vi "VMS_6_Responder.vi"() -> ()   [LabVIEW 2023]
uses:
  <vilib>/rvi/Emulation/niFpgaGetClockAttributes.vi
  <vilib>/rvi/Emulation/niFpgaSctlEmulationGetInTimedLoop.vi
  <vilib>/rvi/Emulation/niFpgaEmulationReportErrorSimple.vi
  <vilib>/rvi/eio/common/nirviEmuTemplateMethod_errors.vi
  <vilib>/eio/utilities/niEioResolveVilibRelativePath.vi
  <vilib>/rvi/interface/RandomDataEmulation/niFpgaRandomDataHandleErrors.vi
  <vilib>/rvi/Emulation/niFpgaProcessEmulError.vi
  <vilib>/rvi/Emulation/niFpgaCriticalErrorInLSC.vi
  <vilib>/rvi/occurrence/nirviWaitOnOccurrenceBase.vi
  <vilib>/eio/EIOMethodNode/EIOMethodNode.xnode
  <vilib>/rvi/DataTransferAndStorage/Container/XNode/niFpgaContainer.xnode
  <vilib>/rvi/interface/RandomDataEmulation/nirviRandomDataFpgaReadWriteTemplate.vi
  <vilib>/eio/EIONode/EIONode.xnode
panel:
  out "Ready":bool
  out "Timeouted":bool
  in  "Period (ms)":u32=5
  out "FIFO full":bool
  out "Stopped":bool
  out "Chassis Temperature":fxp<+/-,32,16>
  out "Ticks":u64
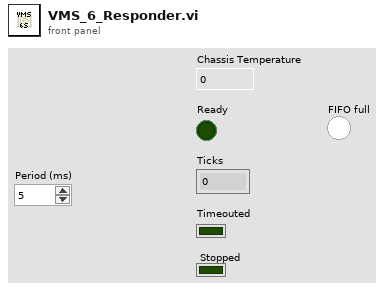
[diagram p1: front panel]
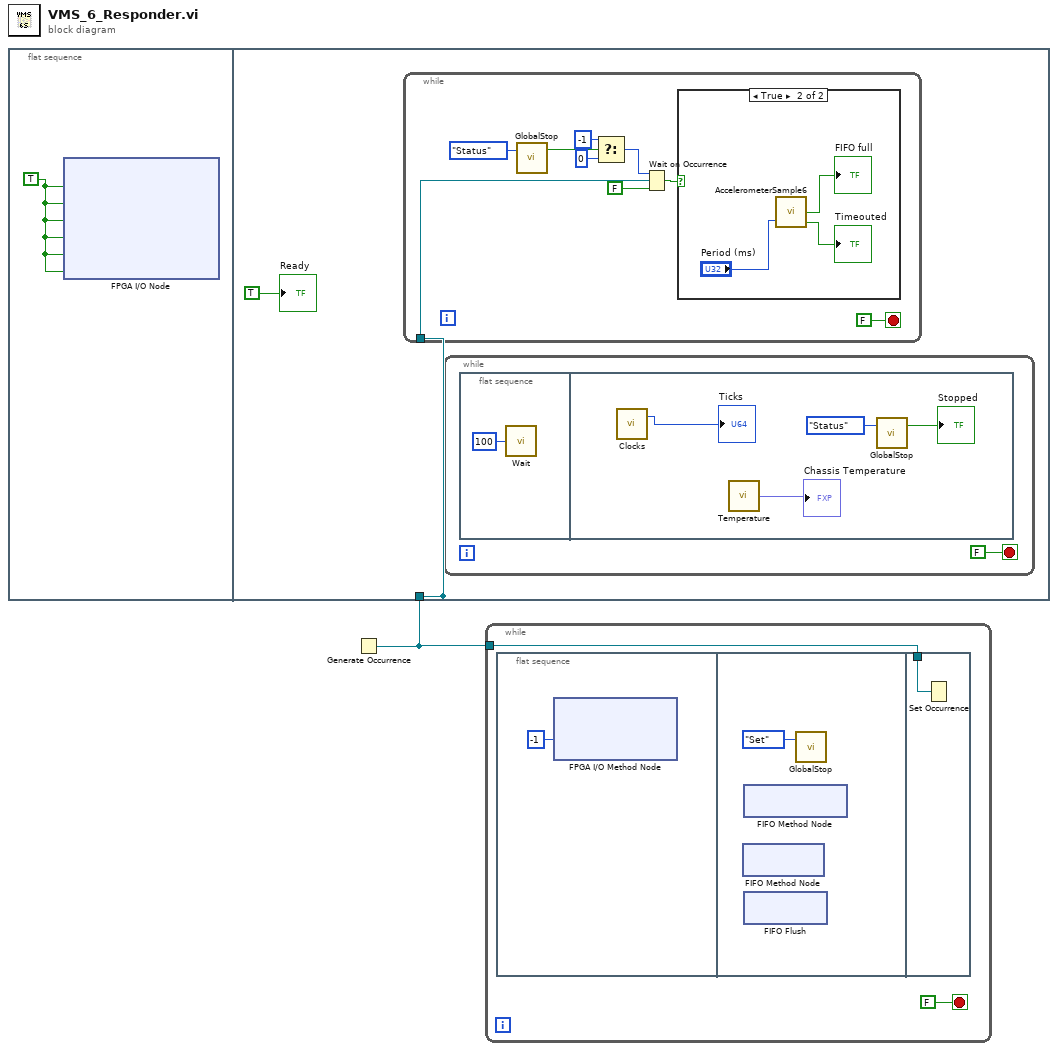
[diagram p0: block diagram]
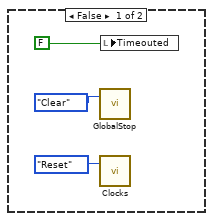
[diagram p2: hidden frame]
diagram:
  n1 = flat-sequence {
    tunnel: w1 -> [w3]
    tunnel: [w3] -> _
    frame #0 {
      w2 = TRUE ("Accelerometer5/Start")
      n2 = xnode "FPGA I/O Node"("Accelerometer1/Start"=w2, "Accelerometer2/Start"=w2, "Accelerometer3/Start"=w2, "Accelerometer4/Start"=w2, "Accelerometer5/Start"=w2, "Accelerometer6/Start"=w2) -> ()  [unwired: 6 in, 6 out]
    }
    frame #1 {
      n3 = while {
        tunnel: w3 -> [w16]
        stop <- FALSE stop-if-true
        n4 = call "GlobalStop.vi"("Enum"=enum16{"Clear", "Set", "Status"}."Status") -> ("Boolean"=w11:bool)  [unwired: 1 in, 1 out]
        n5 = Select(t=-1, s=w11, f=0) -> (s? t:f=w15:i32)
        n6 = Wait on Occurrence(1:FALSE ("ignore previous (T)"), 2:w16, 3:w15) -> (0:w17:bool)
        n7 = case shown="True" w17 {
          frame False {
            n8 = call "GlobalStop.vi"("Enum"=enum16{"Clear", "Set", "Status"}."Clear") -> ()  [unwired: 1 in, 2 out]
            n9 = call "Clocks.vi"("Enum"=enum16{"Reset", "Increment", "Get"}."Reset") -> ()  [unwired: 1 in, 2 out]
            n10 = local write "Timeouted"(FALSE ("Timeouted")) -> ()
          }
          frame True {
            n11 = call "AccelerometerSample6.vi"("Period (ms)"="Period (ms)") -> ("FIFO full"=→"FIFO full":bool, "Timeouted"=→"Timeouted":bool)  [unwired: 1 in, 1 out]
          }
        }
      }
      n12 = while {
        stop <- FALSE stop-if-true
        n13 = flat-sequence {
          frame #0 {
            n14 = call "Wait"("Count(mSec)"=u32 100) -> ()  [unwired: 1 out]
          }
          frame #1 {
            n15 = call "Clocks.vi"() -> ("Clock"=→"Ticks":u64)  [unwired: 2 in, 1 out]
            n16 = call "Temperature.vi"() -> ("Mean temperature"=→"Chassis Temperature":fxp<+/-,32,16>)  [unwired: 1 in]
            n17 = call "GlobalStop.vi"("Enum"=enum16{"Clear", "Set", "Status"}."Status") -> ("Boolean"=→"Stopped":bool)  [unwired: 1 in, 1 out]
          }
        }
      }
      "Ready" <- TRUE ("Ready")
    }
  }
  n18 = Generate Occurrence() -> (w1:refnum<k4>)
  n19 = while {
    tunnel: w1 -> [w26]
    stop <- FALSE stop-if-true
    n20 = flat-sequence {
      tunnel: w26 -> [w30]
      frame #0 {
        n21 = xnode "FPGA I/O Method Node"("Timeout"=-1) -> ()  [unwired: 1 in, 2 out]
      }
      frame #1 {
        n22 = xnode ("FIFO Method Node")() -> ()  [unwired: 1 in, 1 out]
        n23 = xnode ("FIFO Method Node")() -> ()  [unwired: 1 in, 1 out]
        n24 = xnode "FIFO Flush"() -> ()  [unwired: 1 in, 1 out]
        n25 = call "GlobalStop.vi"("Enum"=enum16{"Clear", "Set", "Status"}."Set") -> ()  [unwired: 1 in, 2 out]
      }
      frame #2 {
        n26 = Set Occurrence(w30) -> ()
      }
    }
  }
